vi "Operation UI.vi"(0 "A":dbl, 5 "B":dbl, 7 "Calculate":bool, 9 "DVR In":refnum<data-value>, 11 "Error In":errorcluster, 12 "Stop":refnum<user-event>, 13 "Class Data":refnum<user-event>) -> (4 "C":dbl, 10 "DVR  Out":refnum<data-value>, 15 "Error Out":errorcluster)   [LabVIEW 2019, in "Add.lvclass"]
doc: "The VI contains the addition operation UI that accepts two input numbers and performs addition operation and displays the output when user clicks calculate button"
uses:
  Add.lvclass
  Typedef/User Event Operations.ctl
  Arithemtic Operation/Arithemetic Operation.lvclass
panel:
  # "ADDITION"
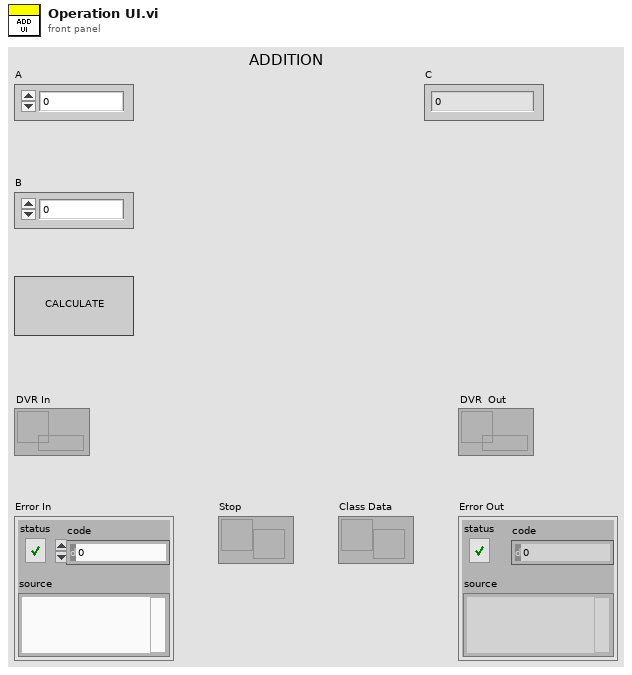
[diagram p1: front panel]
types:
  T1 = typedef "User Event Operations.ctl" = enum16{"Obtain", "Generate", "Release"}
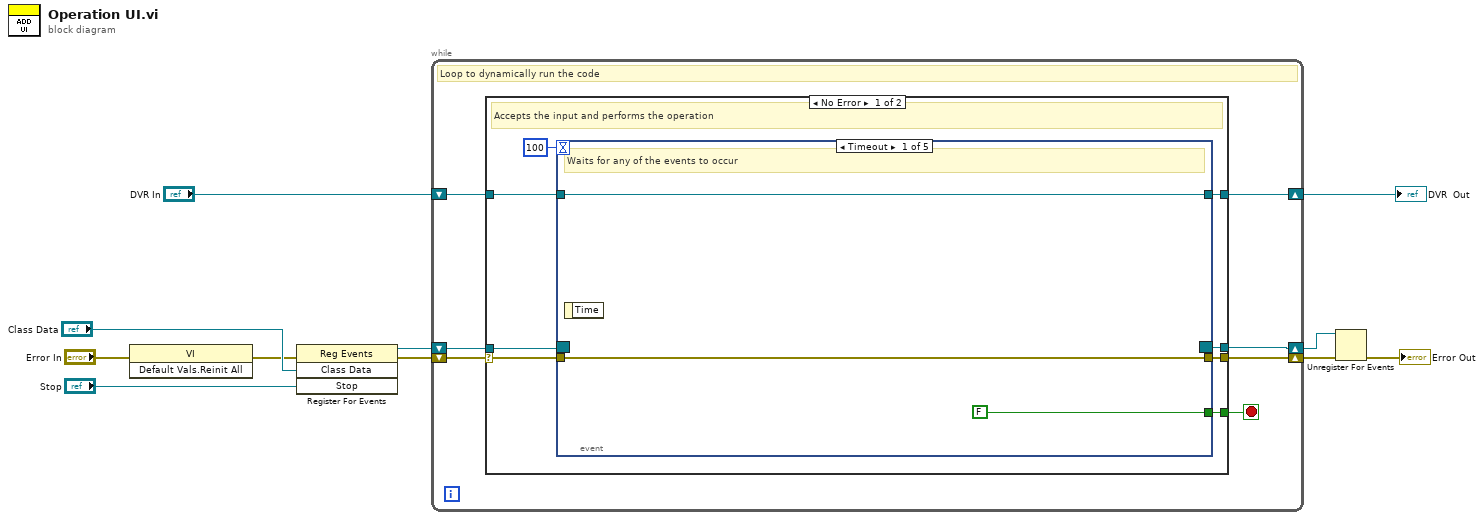
[diagram p0: block diagram]
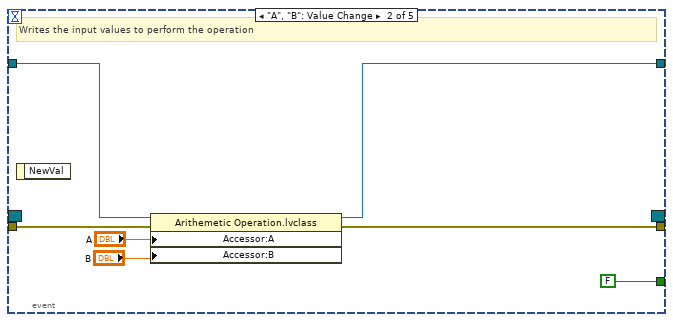
[diagram p2: hidden frame]
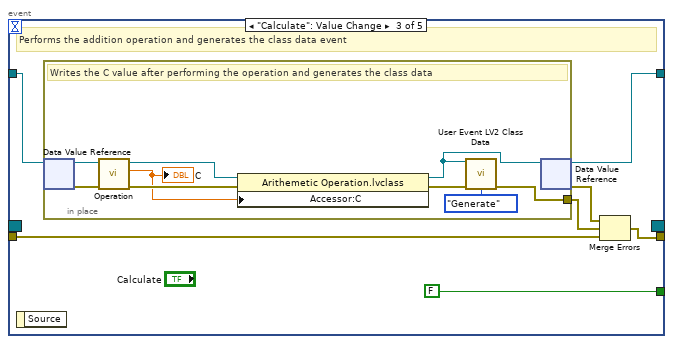
[diagram p3: hidden frame]
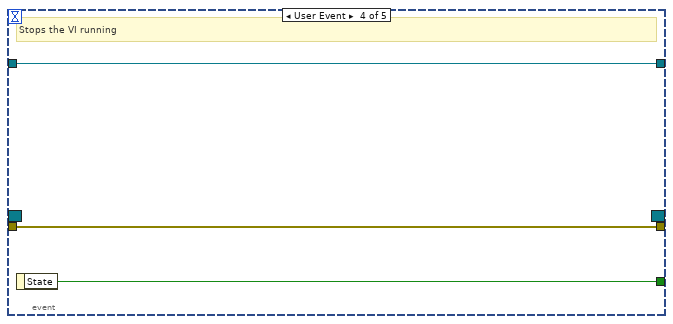
[diagram p4: hidden frame]
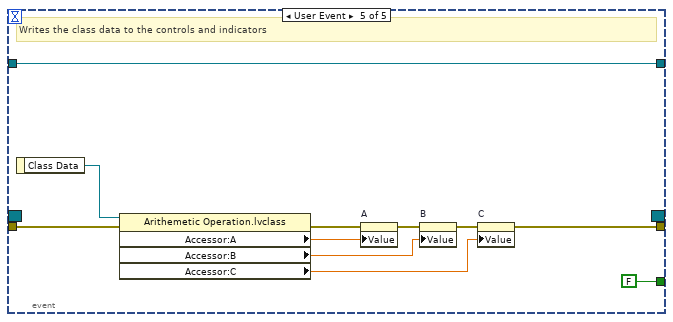
[diagram p5: hidden frame]
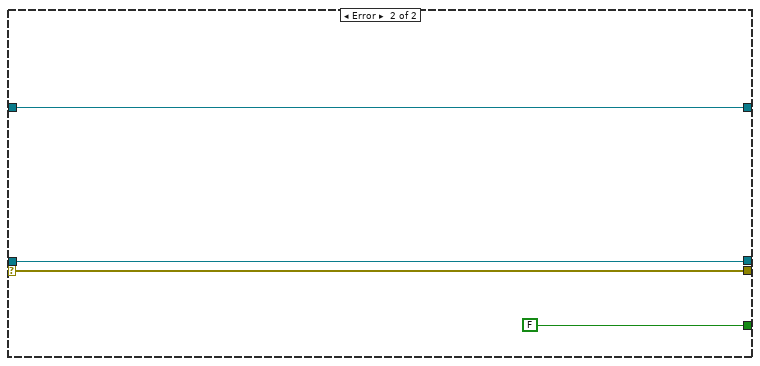
[diagram p6: hidden frame]
diagram:
  n1 = invoke class="VI" method="Default Vals.Reinit All"(error in="Error In") -> (error out=w3:errorcluster)  [unwired: 2 in, 2 out]
  n2 = register-events(error in=w3, "Class Data", "Stop") -> (reference out=w9:refnum<event-registration>, error out=w10:errorcluster)  [unwired: 1 in]
  n3 = while {
    shift-right: [w17] -> w11
    shift-left: w10 -> [w18]
    shift-right: [w15] -> w1
    shift-left: "DVR In" -> [w16]
    shift-right: [w12] -> w6
    shift-left: w9 -> [w14]
    stop <- w13 stop-if-true
    # "Loop to dynamically run the code"
    n4 = case shown="No Error" w18 {
      selector: w18 -> [w24 w70]
      tunnel: [w23 w70] -> w17
      tunnel: [w25 w69] -> w15
      tunnel: w16 -> [w26 w69]
      tunnel: w14 -> [w21 w68]
      tunnel: [w20 w68] -> w12
      tunnel: [w19 FALSE] -> w13
      frame No Error {
        # "Accepts the input and performs the operation"
        n5 = event shown="[0] Timeout" {
          selector: w21 -> [_ _ _ _ _]
          dyn-events: [_ _ _ _ _] -> w20
          timeout: 100 -> [_ _ _ _ _]
          tunnel: [w29 w31 w41 w55 w66] -> w25
          tunnel: w26 -> [w29 w34 w42 w55 w66]
          tunnel: w24 -> [w28 w36 w39 w54 w65]
          tunnel: [w28 w35 w37 w54 w59] -> w23
          tunnel: [FALSE FALSE FALSE w53 FALSE] -> w19
          event Timeout {
            # "Waits for any of the events to occur"
            n6 = event-data() -> ()  [unwired: 1 in, 1 out]
          }
          event "A", "B": Value Change {
            # "Writes the input values to perform the operation"
            n7 = event-data() -> ()  [unwired: 1 in, 1 out]
            n8 = property class="Arithemetic Operation.lvclass"(reference=w34, error in=w36, "Accessor:A"="A", "Accessor:B"="B") -> (reference out=w31:refnum<data-value>, error out=w35:errorcluster)
          }
          event "Calculate": Value Change {
            # "Performs the addition operation and generates the class data event"
            n9 = event-data() -> ()  [unwired: 1 in, 1 out]
            n10 = in-place {
              in-place-border: [w44] -> w38
              # "Writes the C value after performing the operation and generates the class data"
              n11 = in-place-dvr #1(w42) -> (w47:refnum<class "Arithemetic Operation.lvclass">, w46:errorcluster)
              n12 = call-dynamic "Operation.vi"("Error In"=w46, "Arithemetic Operation in"=w47) -> ("Error Out"=w52:errorcluster, "C"=w49:dbl, "Arithemetic Operation out"=w50:refnum<class "Arithemetic Operation.lvclass">)  [unwired: 7 in]
              "C" <- w49
              n13 = property class="Arithemetic Operation.lvclass"(reference=w50, error in=w52, "Accessor:C"=w49) -> (reference out=w45:refnum<class "Arithemetic Operation.lvclass">, error out=w51:errorcluster)
              n14 = call "User Event LV2 Class Data.vi"("Class Data"=w45, "Error In"=w51, "Operation"=User_Event_Operations."Generate") -> ("Error Out"=w44:errorcluster)  [unwired: 11 in, 1 out]
              n15 = in-place-dvr #1(w45) -> (w41:refnum<data-value>, w40:errorcluster)
            }
            n16 = Merge Errors(w40, w38, w39) -> (w37:errorcluster)
          }
          event User Event {
            # "Stops the VI running"
            n17 = event-data() -> ("State"=w53:bool)  [unwired: 1 in]
          }
          event User Event {
            # "Writes the class data to the controls and indicators"
            n18 = event-data() -> ("Class Data"=w62:refnum<class "Arithemetic Operation.lvclass">)  [unwired: 1 in]
            n19 = property class="Arithemetic Operation.lvclass"(reference=w62, error in=w65) -> (error out=w63:errorcluster, "Accessor:A"=w58:dbl, "Accessor:B"=w57:dbl, "Accessor:C"=w56:dbl)  [unwired: 1 out]
            n20 = property on="A" class="DigNum (strict)"(error in=w63, "Value"=w58) -> (error out=w60:errorcluster)  [unwired: 1 in, 1 out]
            n21 = property on="B" class="DigNum (strict)"(error in=w60, "Value"=w57) -> (error out=w61:errorcluster)  [unwired: 1 in, 1 out]
            n22 = property on="C" class="DigNum (strict)"(error in=w61, "Value"=w56) -> (error out=w59:errorcluster)  [unwired: 1 in, 1 out]
          }
        }
      }
      frame Error {
      }
    }
  }
  "DVR  Out" <- w1
  n23 = Unregister For Events(event registration refnum=w6, error in=w11) -> (error out=→"Error Out":errorcluster)
